vi "Aspect Ratio.vi"(10 "Diameter":dbl, 11 "Convex Hull Area":dbl) -> (3 "Score":dbl)   [LabVIEW 2025]
doc: "This VI compares the calculated diameter and convex hull area to compare this shape to a half-hexagon."
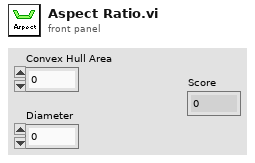
[diagram p1: front panel]
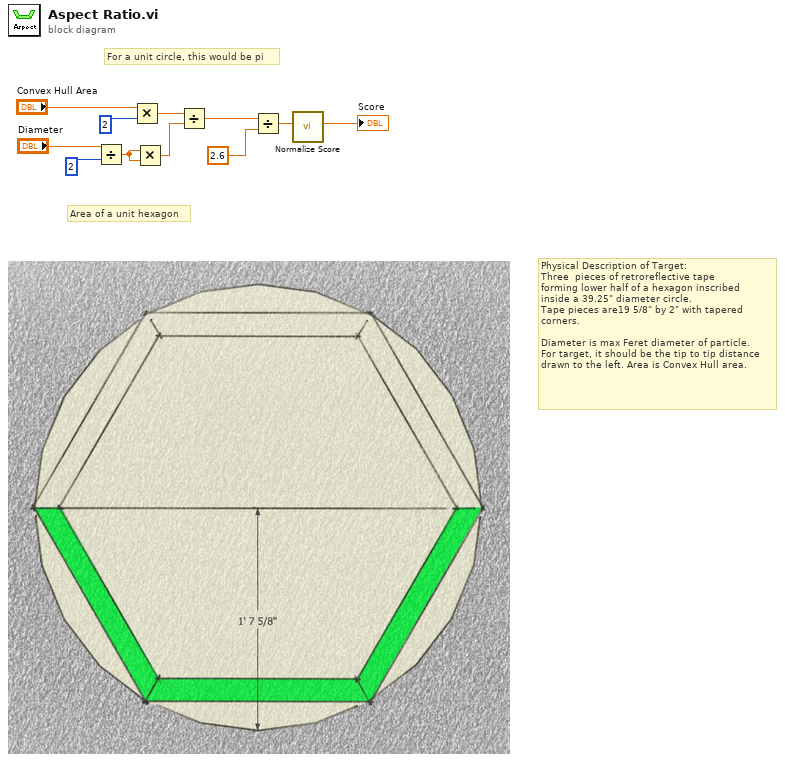
[diagram p0: block diagram]
diagram:
  # "Area of a unit hexagon"
  # "For a unit circle, this would be pi"
  # "Physical Description of Target:\nThree  pieces of retroreflective tape\nforming lower half of a hexagon inscribed\ninside a 39.25\" diameter circle.\nTape pieces are19 5/8\" by 2\" with tapered\ncorners.\n\nDiameter is max Feret diameter of particle.\nFor target, it should be the tip to tip distance\ndrawn to the left. Area is Convex Hull area."
  n1 = Divide(x="Diameter", y=2 ("index")) -> (x/y=w7:dbl)
  n2 = Multiply(x="Convex Hull Area", y=2 ("index")) -> (x*y=w6:dbl)
  n3 = Multiply(x=w7, y=w7) -> (x*y=w5:dbl)
  n4 = Divide(x=w6, y=w5) -> (x/y=w3:dbl)
  n5 = Divide(x=w3, y=2.6 ("index")) -> (x/y=w2:dbl)
  n6 = call "Normalize Score.vi"("Value"=w2) -> ("Score"=→"Score":dbl)  [unwired: 10 in]
